vi "setInternalProcessCommand.vi"(10 "InternalProcessCommand":refnum<user-event>, 11 "UserEvents in":refnum<class "UserEvents.lvclass">) -> (3 "UserEvents out":refnum<class "UserEvents.lvclass">)   [LabVIEW 2016, in "UserEvents.lvclass"]
uses:
  UserEvents.lvclass
  DataTypes/General/ProcessCommandEvent.ctl
  Commands/Command/Command.lvclass
  UserEvents.lvclass/UserEvents.ctl
  DataTypes/General/M1M3SupportGeneral.lvlib
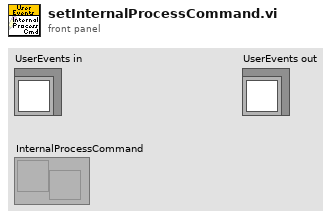
[diagram p1: front panel]
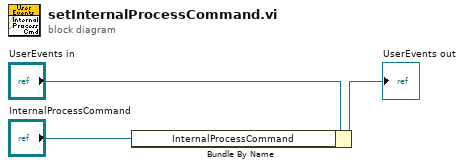
[diagram p0: block diagram]
diagram:
  n1 = Bundle By Name(cluster="UserEvents in", "InternalProcessCommand"="InternalProcessCommand") -> (→"UserEvents out":refnum<class "UserEvents.lvclass">)
